vi "Example.vi"() -> ()   [LabVIEW 2015, in "Mediator.lvlib"]
uses:
  Mediator.lvlib
  Classes/Mediator/Controls/Sequence Return Info.ctl
  Classes/Sequence/Sequence.lvclass
  Example Step One/Example Step One.lvclass
  Classes/Mediator/Mediator.lvclass
  Example Step Two/Example Step Two.lvclass
panel:
  out "Sequence Error Info":T1
  in  "Step One Execution Count":i32
  in  "Stop":bool
  out "error out":errorcluster
  in  "error in (no error)":errorcluster
  in  "Run Step":bool
  in  "Console":string
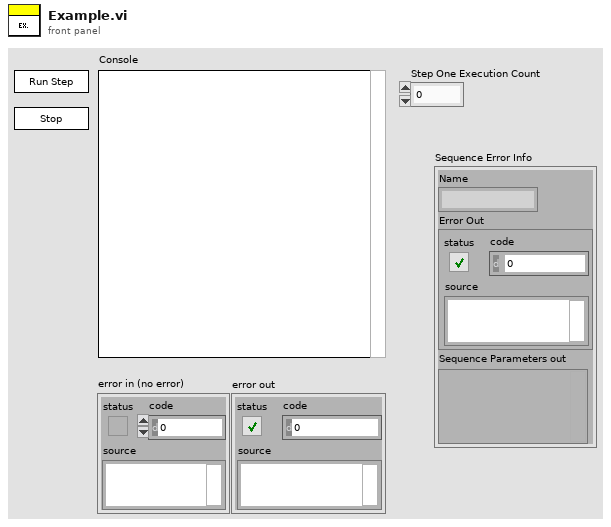
[diagram p1: front panel]
types:
  T1 = typedef "Mediator.lvlib/Sequence.lvclass/Sequence Return Info.ctl" = cluster{"Name":string, "Error Out":errorcluster, "Sequence Parameters out":variant}
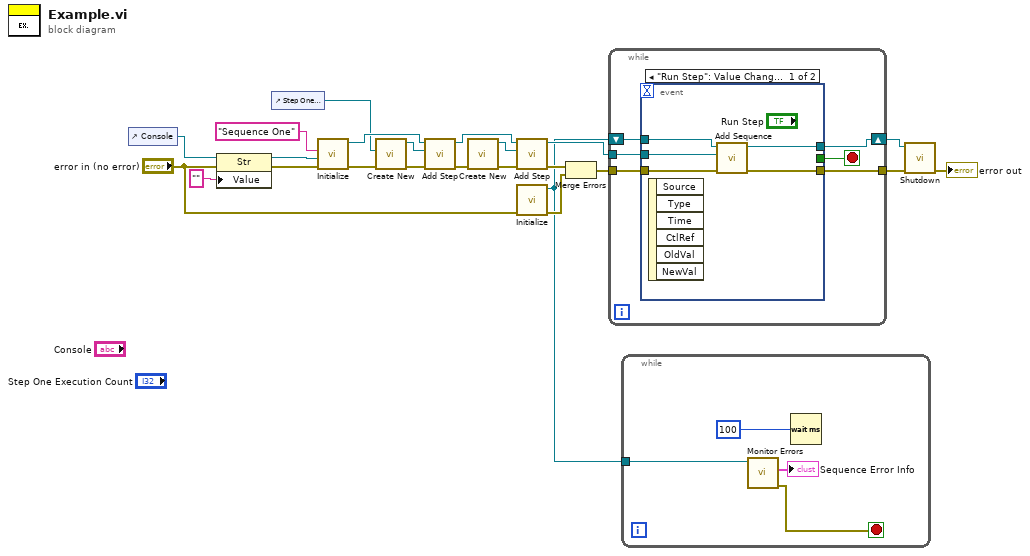
[diagram p0: block diagram]
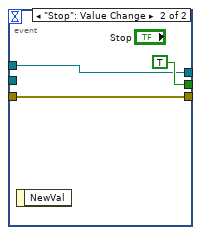
[diagram p2: hidden frame]
diagram:
  n1 = control-ref of="Console"() -> (w11:refnum<vi>)
  n2 = property class="Str"(reference=w11, error in="error in (no error)", "Value"="") -> (reference out=w9:refnum<vi>, error out=w8:errorcluster)
  n3 = control-ref of="Step One Execution Count"() -> (w3:refnum<vi>)
  n4 = call "Initialize.vi"("error in (no error)"=w8, "Parameters In"=w9, "Name"="Sequence One") -> ("error out"=w20:errorcluster, "Sequence out"=w21:refnum<class "Sequence.lvclass">)  [unwired: 7 in]
  n5 = call "Create New.vi"("error in (no error)"=w20, "DigNum Refnum"=w3) -> ("error out"=w19:errorcluster, "Example Step One out"=w1:refnum<class "Example Step One.lvclass">)  [unwired: 8 in]
  n6 = call-dynamic "Add Step.vi"("error in (no error)"=w19, "Step In"=w1, "Sequence in"=w21) -> ("error out"=w14:errorcluster, "Sequence out"=w22:refnum<class "Sequence.lvclass">)  [unwired: 7 in]
  n7 = call "Create New.vi"("error in (no error)"=w14) -> ("error out"=w13:errorcluster, "Example Step One out"=w12:refnum<class "Example Step Two.lvclass">)  [unwired: 9 in]
  n8 = call-dynamic "Add Step.vi"("error in (no error)"=w13, "Step In"=w12, "Sequence in"=w22) -> ("error out"=w4:errorcluster, "Sequence out"=w18:refnum<class "Sequence.lvclass">)  [unwired: 7 in]
  n9 = call "Initialize.vi"("error in (no error)"="error in (no error)") -> ("error out"=w5:errorcluster, "Mediator out"=w2:refnum<class "Mediator.lvclass">)  [unwired: 9 in]
  n10 = Merge Errors(w4, w5) -> (w6:errorcluster)
  n11 = while {
    tunnel: w18 -> [w29]
    tunnel: w6 -> [w27]
    tunnel: [w26] -> w16
    shift-right: [w24] -> w17
    shift-left: w2 -> [w28]
    stop <- w25 stop-if-true
    n12 = event shown="[0] \"Run Step\": Value Change" {
      selector: _ -> [_ _]
      dyn-events: _ -> [_ _]
      timeout: _ -> [_ _]
      tunnel: w29 -> [w33 _]
      tunnel: w28 -> [w34 w35]
      tunnel: w27 -> [w32 w36]
      tunnel: [w31 w36] -> w26
      tunnel: [_ TRUE] -> w25
      tunnel: [w30 w35] -> w24
      event "Run Step": Value Change {
        n13 = event-data() -> ()  [unwired: 1 in, 6 out]
        n14 = call "Add Sequence.vi"("error in (no error)"=w32, "Sequence In"=w33, "Mediator in"=w34) -> ("error out"=w31:errorcluster, "Mediator out"=w30:refnum<class "Mediator.lvclass">)  [unwired: 7 in]
      }
      event "Stop": Value Change {
        n15 = event-data() -> ()  [unwired: 1 in, 1 out]
      }
    }
  }
  n16 = while {
    tunnel: w2 -> [w39]
    stop <- w40 stop-if-true
    n17 = call "Monitor Errors.vi"("Mediator in"=w39) -> ("error out"=w40:errorcluster, "Sequence Error Info"=→"Sequence Error Info":T1)  [unwired: 8 in, 1 out]
    n18 = Wait (ms)(milliseconds to wait=100) -> ()  [unwired: 1 out]
  }
  n19 = call "Shutdown.vi"("error in (no error)"=w16, "Mediator in"=w17) -> ("error out"=→"error out":errorcluster)  [unwired: 9 in]
